vi "L or R.vi"   [LabVIEW 2020]
uses:
  Robot Global Data.vi
  RX.vi
  LX.vi
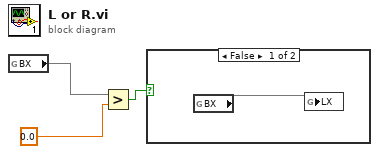
[diagram p0: block diagram]
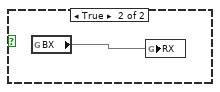
[diagram p2: hidden frame]
diagram:
  n1 = global read "Robot Global Data.vi" "BX"() -> (w3)
  n2 = Greater?(x=w3, y=0.0 ("x")) -> (0:w1:bool)
  n3 = case shown="False" w1 {
    frame False {
      n4 = global read "Robot Global Data.vi" "BX"() -> (w4)
      n5 = global write "LX.vi" "LX"(w4) -> ()
    }
    frame True {
      n6 = global read "Robot Global Data.vi" "BX"() -> (w5)
      n7 = global write "RX.vi" "RX"(w5) -> ()
    }
  }
